vi "02 WriteOff.vi"(8 "error in (no error)":errorcluster caption="错误输入（无错误）", 11 "TCPClientClass 输入":refnum<class "TCPClientClass.lvclass">) -> (0 "error out":errorcluster caption="错误输出", 3 "TCPClientClass 输出":refnum<class "TCPClientClass.lvclass">)   [LabVIEW 2019, in "TCPClientClass.lvclass"]
uses:
  TCPClientClass.lvclass
  TCPClientClass.lvclass/TCPClientClass.ctl
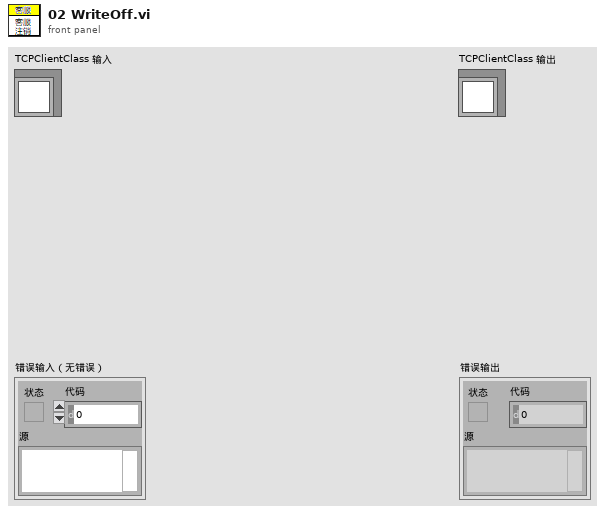
[diagram p1: front panel]
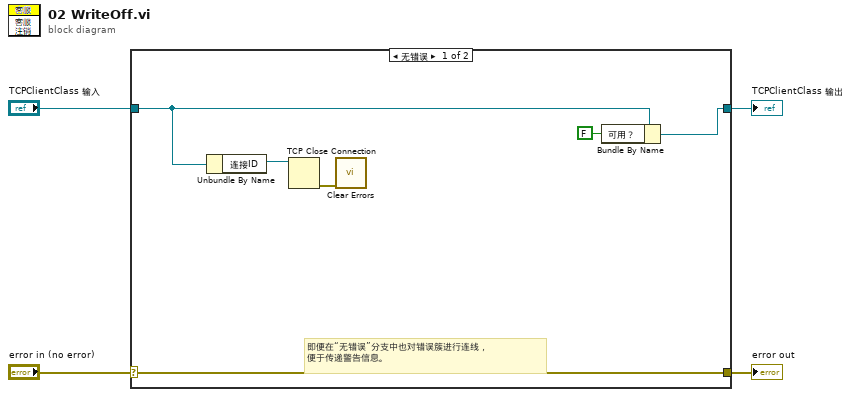
[diagram p0: block diagram]
diagram:
  n1 = case shown="无错误" "error in (no error)" {
    selector: "error in (no error)" -> [w10 w12]
    tunnel: [w10 w12] -> w3
    tunnel: [w5 w11] -> w1
    tunnel: "TCPClientClass 输入" -> [w7 w11]
    frame No Error {
      # "即便在“无错误”分支中也对错误簇进行连线，\n便于传递警告信息。"
      n2 = Unbundle By Name(w7) -> ("连接ID"=w9:refnum<k5>)
      n3 = TCP Close Connection(connection ID=w9) -> (error out=w8:errorcluster)  [unwired: 2 in, 1 out]
      n4 = call <vilib>:"Clear Errors.vi"("error in (no error)"=w8) -> ()  [unwired: 5 in, 2 out]
      n5 = Bundle By Name(cluster=w7, "可用？"=FALSE) -> (w5:refnum<class "TCPClientClass.lvclass">)
    }
    frame Error {
    }
  }
  "error out" <- w3
  "TCPClientClass 输出" <- w1
